vi "Create Resources.vi"(0 "clip resources in":T1, 5 "address space size":u32, 7 "address space uid":u16) -> (4 "niInstr AXI4-Lite - FXP32 address - fxp32 data v1 FPGA out":refnum<class "niInstr AXI4-Lite - FXP32 Address - FXP32 Data v1 FPGA.lvclass">)   [LabVIEW 2015, in "niInstr AXI4-Lite - FXP32 Address - FXP32 Data v1 FPGA.lvclass"]
doc: "Creates a new FPGA resource with 32-bit Fixed Point Address and 32-bit Fixed Point Data.\n\n<b>Do not place this VI into a case structure or it will not compile correctly!</b>\n\n<B>Input Parameters</B>\n\n<B>clip resources in</B> is a collection of CLIP signals to use when creating the resource.\n\n<B>address space size</B> is the size of the address space, in bytes.\n\n<B>address space uid</B> is the globally unique identifier for the address space.\n\n<B>Output Parameters</B>\n\n<B>niInstr AXI4-Lite - FXP32 address - fxp32 data v1 FPGA out</B> passes a reference to the class to the next VI."
uses:
  <instrlib>/_niInstr/CLIP Adapters/v1/FPGA/AXI4-Lite/FXP32 Address - FXP32 Data/niInstr AXI4-Lite - FXP32 Address - FXP32 Data v1 FPGA.lvclass
  <instrlib>/_niInstr/CLIP Adapters/v1/FPGA/AXI4-Lite/FXP32 Address - FXP32 Data/Public/CLIP Resources.ctl
  <instrlib>/_niInstr/CLIP Adapters/v1/FPGA/AXI4-Lite/FXP32 Address - FXP32 Data/niInstr AXI4-Lite - FXP32 Address - FXP32 Data v1 FPGA.lvclass/niInstr AXI4-Lite - FXP32 Address - FXP32 Data v1 FPGA.ctl
  <instrlib>/_niInstr/CLIP Adapters/v1/FPGA/AXI4-Lite/Address Space/niInstr AXI4-Lite Address Space v1 FPGA.lvclass
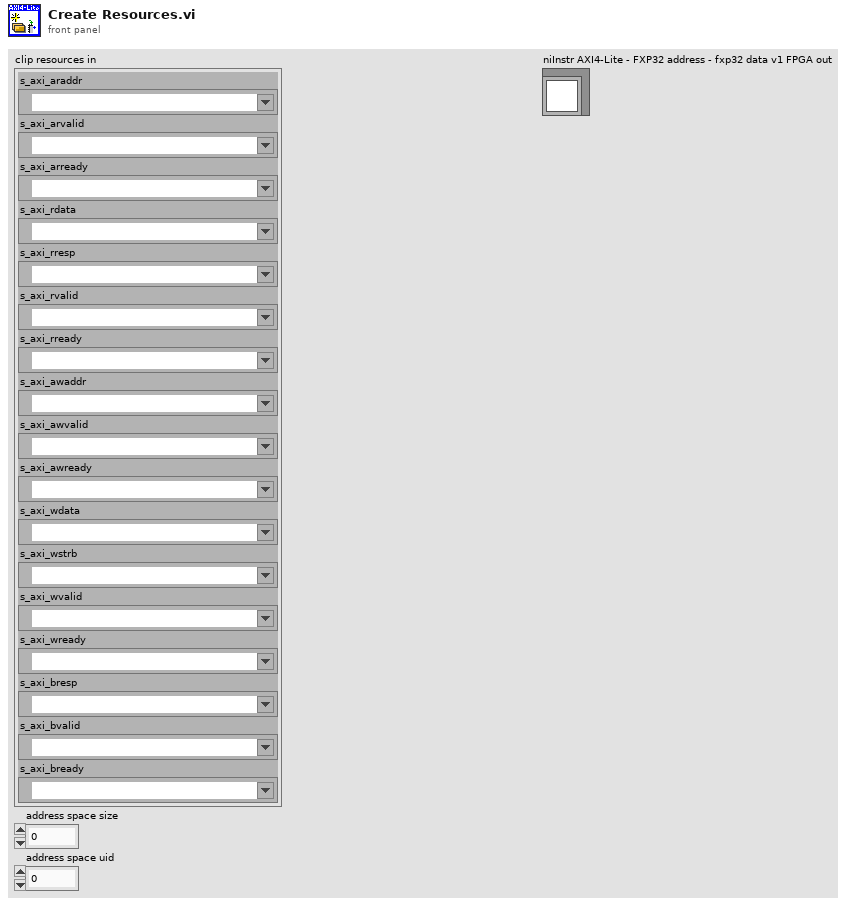
[diagram p1: front panel]
types:
  T1 = typedef "niInstr AXI4-Lite - FXP32 Address - FXP32 Data v1 FPGA.lvclass/CLIP Resources.ctl" = cluster{"s_axi_araddr":refnum<k21>, "s_axi_arvalid":refnum<k21>, "s_axi_arready":refnum<k21>, "s_axi_rdata":refnum<k21>, "s_axi_rresp":refnum<k21>, "s_axi_rvalid":refnum<k21>, "s_axi_rready":refnum<k21>, "s_axi_awaddr":refnum<k21>, "s_axi_awvalid":refnum<k21>, "s_axi_awready":refnum<k21>, "s_axi_wdata":refnum<k21>, "s_axi_wstrb":refnum<k21>, "s_axi_wvalid":refnum<k21>, "s_axi_wready":refnum<k21>, "s_axi_bresp":refnum<k21>, "s_axi_bvalid":refnum<k21>, "s_axi_bready":refnum<k21>}
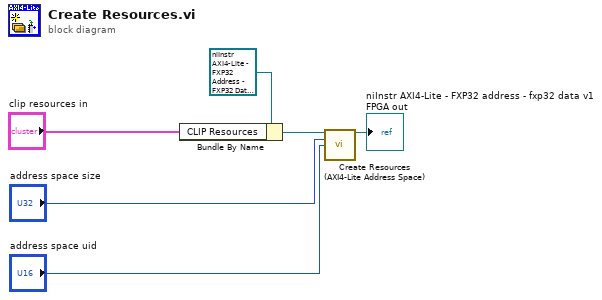
[diagram p0: block diagram]
diagram:
  n1 = Bundle By Name(cluster=refnum<class "niInstr AXI4-Lite - FXP32 Address - FXP32 Data v1 FPGA.lvclass"> refnum ("AXI4-Lite Address Space U32 - 1 spc.lvclass"), "CLIP Resources"="clip resources in") -> (w2:refnum<class "niInstr AXI4-Lite - FXP32 Address - FXP32 Data v1 FPGA.lvclass">)
  n2 = call <instrlib>:"Create Resources (AXI4-Lite Address Space).vi"("niInstr AXI4-Lite address space v1 FPGA in"=w2, "address space size"="address space size", "address space uid"="address space uid") -> ("niInstr AXI4-Lite address space v1 FPGA out"=→"niInstr AXI4-Lite - FXP32 address - fxp32 data v1 FPGA out":refnum<class "niInstr AXI4-Lite - FXP32 Address - FXP32 Data v1 FPGA.lvclass">)  [unwired: 12 in]
